vi "subHamamatsu_DefineROI.vi"(5 "ROI selection":u16(ring) items=["Full ROI", "Central quad", "Confocal"], 7 "ROI define":bool, 11 "ROI cursor":T1={"Bin"=2, "ROI"={"x offset"=256, "y offset"=256, "x width"=512, "y width"=512}} caption="ROI" {"ROI"."x offset" min=1 max=512 step=1; "ROI"."y offset" min=1 max=512 step=1; "ROI"."x width" min=1 max=512 step=1; "ROI"."y width" min=1 max=512 step=1; "Bin" items=["1x1"=1, "2x2"=2, "4x4"=4]}) -> (3 "ROI out":T1={"Bin"=2, "ROI"={"x offset"=256, "y offset"=256, "x width"=512, "y width"=512}} caption="ROI" {"ROI"."x offset" min=1 max=512 step=1; "ROI"."y offset" min=1 max=512 step=1; "ROI"."x width" min=1 max=512 step=1; "ROI"."y width" min=1 max=512 step=1; "Bin" items=["1x1"=1, "2x2"=2, "4x4"=4]})   [LabVIEW 2015]
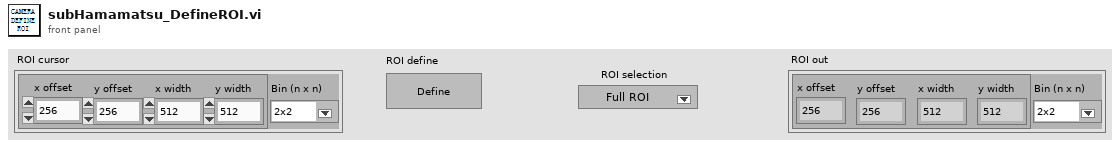
[diagram p1: front panel]
types:
  T1 = cluster{"Bin":u16, "ROI":cluster{"x offset":i32, "y offset":i32, "x width":i32, "y width":i32}}
  T2 = cluster{"x offset":i32, "y offset":i32, "x width":i32, "y width":i32}
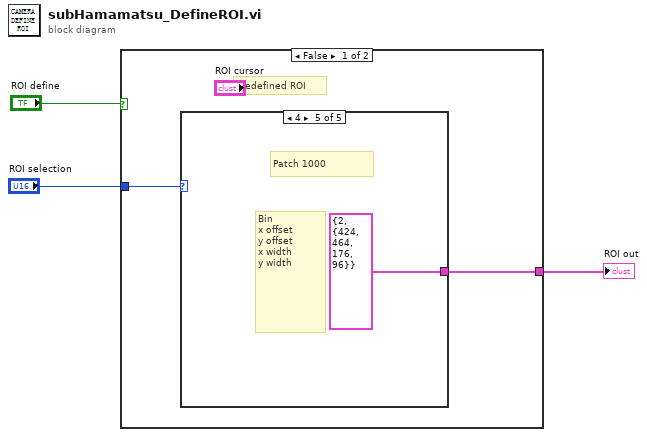
[diagram p0: block diagram]
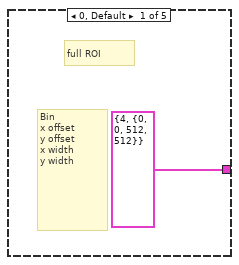
[diagram p2: hidden frame]
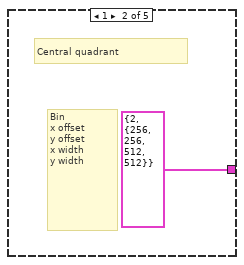
[diagram p3: hidden frame]
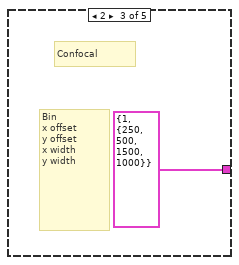
[diagram p4: hidden frame]
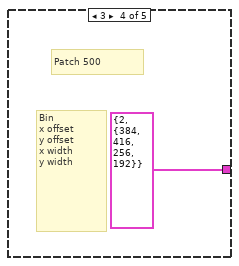
[diagram p5: hidden frame]
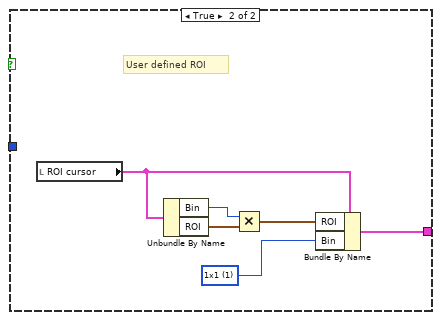
[diagram p6: hidden frame]
diagram:
  n1 = case shown="False" "ROI define" {
    tunnel: [w5 w12] -> w1
    tunnel: "ROI selection" -> [w4 _]
    frame False {
      # "Predefined ROI"
      n2 = case shown="4" w4 {
        tunnel: [T1 {"Bin"=4, "ROI"={"x offset"=0, "y offset"=0, "x width"=512, "y width"=512}} ("ROI cursor 2") T1 {"Bin"=2, "ROI"={"x offset"=256, "y offset"=256, "x width"=512, "y width"=512}} ("ROI cursor 2") T1 {"Bin"=1, "ROI"={"x offset"=250, "y offset"=500, "x width"=1500, "y width"=1000}} ("ROI cursor 2") T1 {"Bin"=2, "ROI"={"x offset"=384, "y offset"=416, "x width"=256, "y width"=192}} ("ROI cursor 2") T1 {"Bin"=2, "ROI"={"x offset"=424, "y offset"=464, "x width"=176, "y width"=96}} ("ROI cursor 2")] -> w5
        frame 0, Default {
          # "Bin\nx offset\ny offset\nx width\ny width"
          # "full ROI"
        }
        frame 1 {
          # "Bin\nx offset\ny offset\nx width\ny width"
          # "Central quadrant"
        }
        frame 2 {
          # "Bin\nx offset\ny offset\nx width\ny width"
          # "Confocal"
        }
        frame 3 {
          # "Bin\nx offset\ny offset\nx width\ny width"
          # "Patch 500"
        }
        frame 4 {
          # "Bin\nx offset\ny offset\nx width\ny width"
          # "Patch 1000"
        }
      }
    }
    frame True {
      w11 = u16 1 items=["1x1"=1, "2x2"=2, "4x4"=4] ("Bin (n x n)")
      # "User defined ROI"
      n3 = local read "ROI cursor"() -> (w13:T1)
      n4 = Unbundle By Name(w13) -> ("Bin"=w16:u16, "ROI"=w15:T2)
      n5 = Multiply(x=w16, y=w15) -> (x*y=w14:T2)
      n6 = Bundle By Name(cluster=w13, "ROI"=w14, "Bin"=w11) -> (w12:T1)
    }
  }
  "ROI out" <- w1
